vi "ReadTree.vi"(8 "error in":errorcluster, 10 "root":T1, 11 "repository in":refnum<class "NISE_CEF_Repository.lvclass">) -> (0 "error out":errorcluster, 3 "repository out":refnum<class "NISE_CEF_Repository.lvclass">)   [LabVIEW 2013, in "NISE_CEF_Repository.lvclass"]
doc: "Transfers information between the repo and the tree control nodes. This should be called before custom views are launched or saving to disk."
uses:
  NISE_CEF_Repository.lvclass
  Node/NodeRef.ctl
  Node/NISE_CEF_Node.lvclass
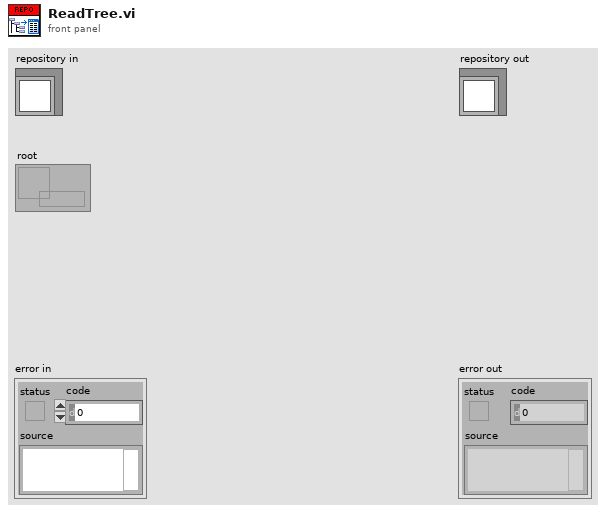
[diagram p1: front panel]
types:
  T1 = typedef "NISE_CEF_Node.lvclass/NodeRef.ctl" = refnum<data-value>
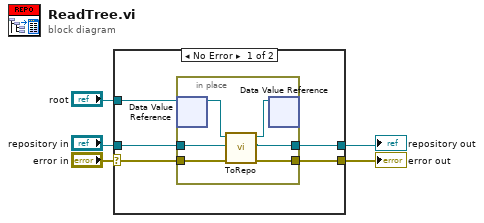
[diagram p0: block diagram]
diagram:
  n1 = case shown="No Error" "error in" {
    selector: "error in" -> [w6 w18]
    tunnel: [w10 w18] -> w4
    tunnel: [w8 w17] -> w2
    tunnel: "repository in" -> [w9 w17]
    tunnel: "root" -> [w7 _]
    frame No Error {
      n2 = in-place {
        in-place-border: w6 -> [w14]
        in-place-border: [w13] -> w10
        in-place-border: w9 -> [w12]
        in-place-border: [w11] -> w8
        n3 = in-place-dvr #1(w7) -> (w16:refnum<class "NISE_CEF_Node.lvclass">)  [unwired: 1 out]
        n4 = call-dynamic "ToRepo.vi"("error in"=w14, "repository in"=w12, "node in"=w16) -> ("error out"=w13:errorcluster, "repository out"=w11:refnum<class "NISE_CEF_Repository.lvclass">, "node out"=w15:refnum<class "NISE_CEF_Node.lvclass">)  [unwired: 6 in]
        n5 = in-place-dvr #1(w15) -> ()  [unwired: 2 out]
      }
    }
    frame Error {
    }
  }
  "error out" <- w4
  "repository out" <- w2
